vi "CmsInitialize.vi"(8 "error in (no error)":errorcluster) -> (0 "error out":errorcluster, 3 "Qbus out":refnum<class "Qbus.lvclass">)   [LabVIEW 2017]
uses:
  <vilib>/addons/Qbus/Qbus.lvclass
  <vilib>/addons/TraceLogger/TraceLogger.lvlib
  <vilib>/addons/SystemInfoProcess/SystemInfoProcess.lvlib
  <vilib>/addons/InsightCM/Utilities/GlobalConfiguration/GlobalConfiguration.lvlib
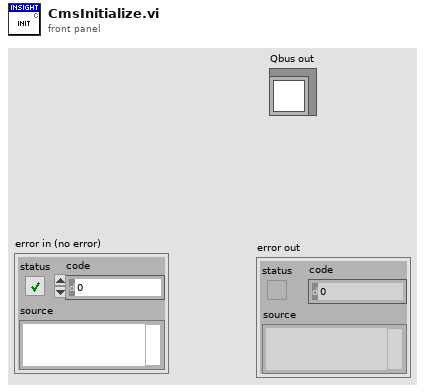
[diagram p1: front panel]
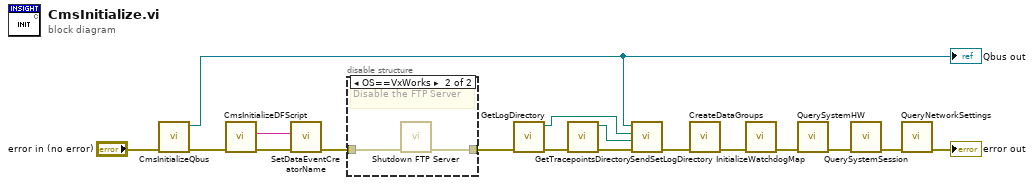
[diagram p0: block diagram]
diagram:
  n1 = call <vilib>:"CmsInitializeQbus.vi"("error in (no error)"="error in (no error)") -> ("error out"=w14:errorcluster, "Qbus out"=w15:refnum<class "Qbus.lvclass">)  [unwired: 9 in]
  "Qbus out" <- w15
  n2 = call <vilib>:"CmsInitializeDFScript.vi"("error in (no error)"=w14) -> ("error out"=w3:errorcluster, "data event creator"=w1:string)  [unwired: 9 in]
  n3 = call <vilib>:"SetDataEventCreatorName.vi"("error in (no error)"=w3, "data event creator"=w1) -> ("error out"=w2:errorcluster)  [unwired: 9 in]
  n4 = disable-structure shown="OS==VxWorks" {
    disable-tunnel: [w18 w20] -> w10
    disable-tunnel: w2 -> [w18 w19]
    frame condition #0 (active) {
    }
    frame condition #1 {
      # "Disable the FTP Server"
      n5 = call <vilib>:"Shutdown FTP Server.vi"("error in (no error)"=w19) -> ("error out"=w20:errorcluster)  [unwired: 10 in]
    }
  }
  n6 = call <vilib>:"GetLogDirectory.vi"("error in (no error)"=w10) -> ("error out"=w6:errorcluster, "log dir"=w9:path)  [unwired: 9 in]
  n7 = call <vilib>:"GetTracepointsDirectory.vi"("error in (no error)"=w6) -> ("error out"=w4:errorcluster, "application directory"=w5:path)  [unwired: 9 in]
  n8 = call <vilib>:"SendSetLogDirectory.vi"("error in (no error)"=w4, "tracpoint directory"=w5, "log directory"=w9, "qbus in"=w15) -> ("error out"=w16:errorcluster)  [unwired: 6 in, 1 out]
  n9 = call <vilib>:"CreateDataGroups.vi"("error in (no error)"=w16) -> ("error out"=w8:errorcluster)  [unwired: 10 in]
  n10 = call <vilib>:"InitializeWatchdogMap.vi"("error in (no error)"=w8) -> ("error out"=w7:errorcluster)  [unwired: 10 in]
  n11 = call <vilib>:"QuerySystemHW.vi"("error in (no error)"=w7) -> ("error out"=w13:errorcluster)  [unwired: 10 in]
  n12 = call <vilib>:"QuerySystemSession.vi"("error in (no error)"=w13) -> ("error out"=w12:errorcluster)  [unwired: 10 in]
  n13 = call <vilib>:"QueryNetworkSettings.vi"("error in (no error)"=w12) -> ("error out"=→"error out":errorcluster)  [unwired: 10 in]
